vi "Load Test Executive.vi"(4 "Compatibility Helper":refnum<class "ICompatibility Helper.lvclass">, 5 "Path Builder":refnum<class "IPath Builder.lvclass">, 6 "File Path":path, 7 "Persistence in":refnum<class "IPersist.lvclass">, 8 "error in (no error)":errorcluster, 11 "Test Executive in":refnum<class "Test Executive.lvclass">) -> (0 "error out":errorcluster, 3 "Test Executive out":refnum<class "Test Executive.lvclass">)   [LabVIEW 2019, in "Test Executive.lvlib" / "Test Executive.lvclass"]
uses:
  <vilib>/gpm_packages/@cs/test-executive/Source/Test Executive/TestExecutive/Test Executive.lvclass
  <vilib>/gpm_packages/@cs/persistence/source/IPersist/IPersist.lvclass
  <vilib>/gpm_packages/@cs/test-executive/Source/Path Builder/IPath Builder/IPath Builder.lvclass
  <vilib>/gpm_packages/@cs/test-executive/Source/Compatibility Helper/ICompatibility Helper.lvclass
  <vilib>/gpm_packages/@cs/linked-list/Source/Linked List/Linked List/Linked List.lvclass
  C:/Program Files/National Instruments/LabVIEW 2019/vi.lib/gpm_packages/@cs/linked-list/Source/Linked List/ILinkedList/ILinked List.lvclass
  <vilib>/gpm_packages/@cs/test-executive/Source/Test Executive/TestExecutive/Test Executive.lvclass/Test Executive.ctl
  <vilib>/gpm_packages/@cs/test-executive/Source/Test Executive/Executioner/Executioner.lvclass
  <vilib>/gpm_packages/@cs/linked-list/Source/Linked List/Linked List Ref/Linked List Ref.lvclass
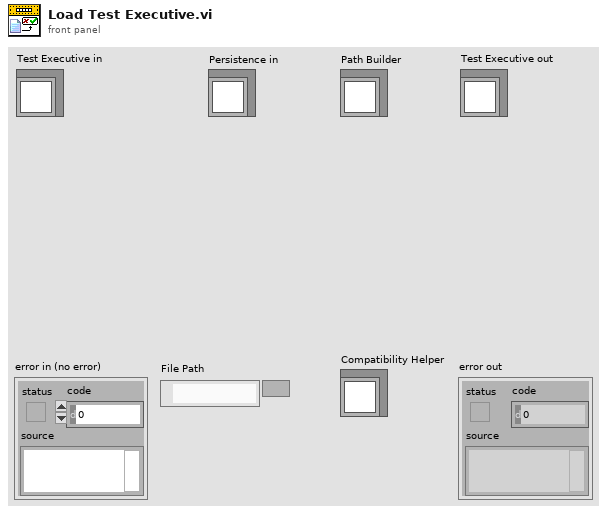
[diagram p1: front panel]
types:
  T1 = enum16{"open", "replace", "create", "open or create", "replace or create", "replace or create with confirmation"}
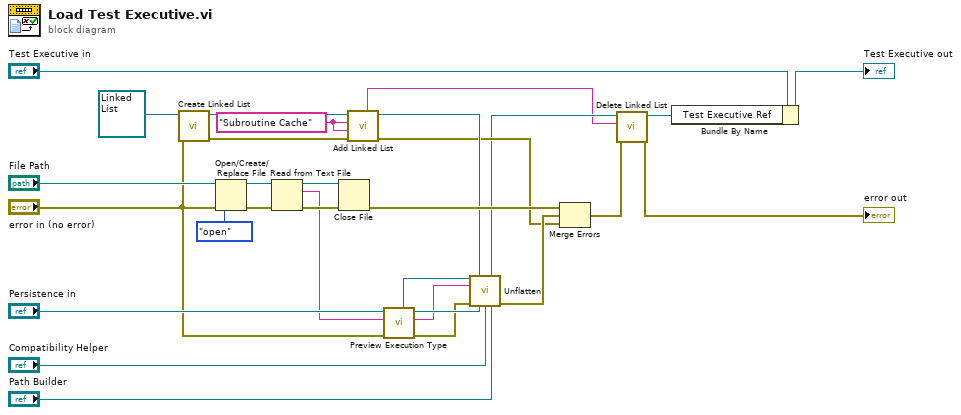
[diagram p0: block diagram]
diagram:
  w6 = "Subroutine Cache" ("Name")
  n1 = call <vilib>:"Create Linked List.vi"("error in (no error)"="error in (no error)", "Linked List"=refnum<class "Linked List.lvclass"> refnum ("Linked Lists.lvlib:Linked List.lvclass")) -> ("error out"=w8:errorcluster, "Linked List Ref"=w10:refnum<data-value>)  [unwired: 8 in]
  n2 = Open/Create/Replace File(file path (use dialog)="File Path", error in="error in (no error)", operation (0:open)=T1."open") -> (refnum out=w25:refnum<file>, error out=w27:errorcluster)  [unwired: 3 in, 1 out]
  n3 = Read from Text File(file (use dialog)=w25, error in=w27) -> (refnum out=w26:refnum<file>, text=w14:string, error out=w28:errorcluster)  [unwired: 2 in, 1 out]
  n4 = Close File(refnum=w26, error in=w28) -> (error out=w23:errorcluster)  [unwired: 1 out]
  n5 = call <vilib>:"Add Linked List.vi"("error in (no error)"=w8, "Linked List ID"=w6, "Name"=w6, "Linked List Ref"=w10) -> ("error out"=w7:errorcluster, "Linked List Ref out"=w9:refnum<data-value>, "Linked List ID out"=w1:string)  [unwired: 4 in, 1 out]
  n6 = call <vilib>:"Preview Execution Type.vi"("error in (no error)"="error in (no error)", "Flattened Linked List"=w14, "IPersist in"="Persistence in") -> ("error out"=w15:errorcluster, "Flattened Linked List out"=w13:string, "IPersist out"=w18:refnum<class "IPersist.lvclass">, "Execution Type"=w16:refnum<class "Executioner.lvclass">)  [unwired: 4 in, 1 out]
  n7 = call-dynamic "Unflatten.vi"("Executioner in"=w16, "Linked List Ref"=w9, "Flattened Test Executive"=w13, "error in (no error)"=w15, "Persistence in"=w18, "Compatibility Helper"="Compatibility Helper", "Path Builder"="Path Builder") -> ("Linked List Ref out"=w5:refnum<data-value>, "error out"=w21:errorcluster)  [unwired: 6 in, 1 out]
  n8 = Merge Errors(w23, w21, w7) -> (w3:errorcluster)
  n9 = call <vilib>:"Delete Linked List.vi"("error in (no error)"=w3, "Linked List ID"=w1, "Linked List Ref"=w5) -> ("error out"=→"error out":errorcluster, "Linked List Ref out"=w4:refnum<data-value>)  [unwired: 7 in]
  n10 = Bundle By Name(cluster="Test Executive in", "Test Executive Ref"=w4) -> (→"Test Executive out":refnum<class "Test Executive.lvclass">)
